vi "M01 Wind Turbine - Dahai.vi"(11 "NXT/EV3":T1) -> (3 "EV3 out":T1)   [LabVIEW 2016]
uses:
  <vilib>/NXT/Subs/LVHSConnector.ctl
  <vilib>/NXT/LegoClasses/BrickReference/BrickReference.lvclass
  <vilib>/NXT/Block Support/NXT_InputPort.ctl
  <vilib>/NXT/Block Support/NXT_OutputPort.ctl
  <vilib>/NXT/Dual Mode Library/Waits/Wait_Num(msec).vi
  <vilib>/NXT/NXTIO Xnodes/NXTIONodeSubVIs/NXTMotorRunDistance.vi
  <vilib>/NXT/NXTIO Xnodes/AddressXNode/NXTIOAddress.xnode
  <vilib>/NXT/NXTIO Xnodes/NXTIOXNode/NXTIO.xnode
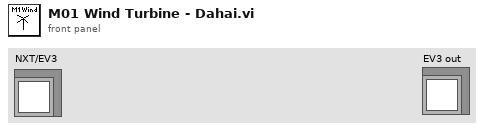
[diagram p1: front panel]
types:
  T1 = typedef "LVHSConnector.ctl" = refnum<class "BrickReference.lvclass">
  T2 = typedef "NXT_OutputPort.ctl" = u8
  T3 = typedef "NXT_InputPort.ctl" = u32
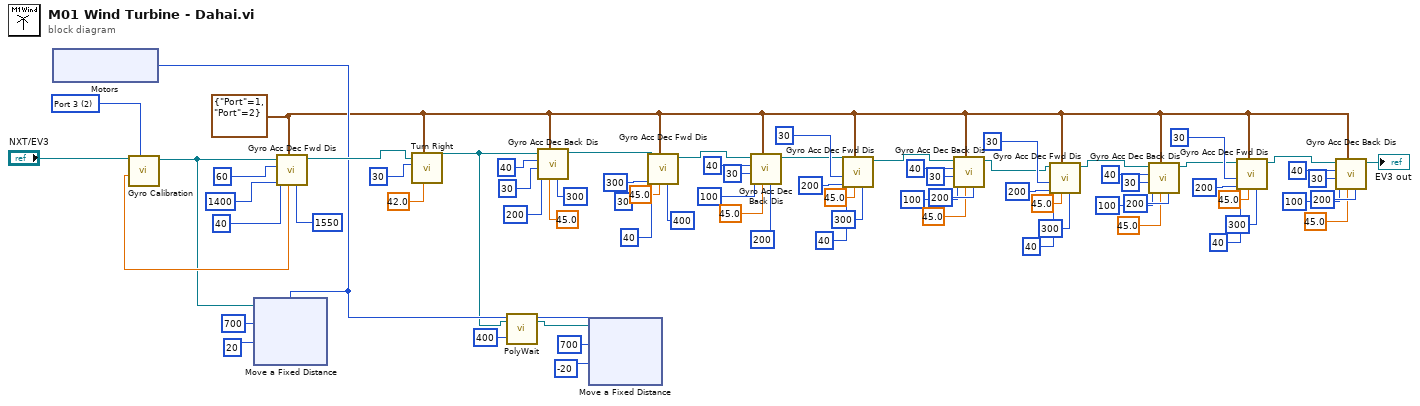
[diagram p0: block diagram]
diagram:
  w2 = cluster{"Port":T2, "Port":T2} {"Port"=1, "Port"=2} ("Motor")
  w74 = T3 2 items=["Port 1", "Port 2", "Port 3", "Port 4"] ("Port (Port 1)")
  n1 = xnode "Motors"() -> ("Motor"=w19:T2)
  n2 = call "Gyro Calibration.vi"("Port (Port 1)"=w74, "NXT/EV3"="NXT/EV3") -> ("Degrees"=w73:sgl, "NXT/EV3"=w23:T1)  [unwired: 5 in, 1 out]
  n3 = xnode "Move a Fixed Distance"("Speed 1"=i8 20, "Distance 1"=700, "Motors"=w19, "NXT/EV3"=w23) -> ()  [unwired: 1 out]
  n4 = call "Gyro Acc Dec Fwd Dis.vi"("Stop rotation"=1550, "Ini. Degrees"=w73, "Motor"=w2, "Threshold to De-acc"=1400, "De-acc"=40, "Acc"=60, "EV3 in"=w23) -> ("EV3 out"=w27:T1)  [unwired: 4 in]
  n5 = call "Turn Right.vi"("Turning angle"=sgl 42.0, "Motor"=w2, "Motor B (right)"=i8 30, "EV3 in"=w27) -> ("EV3 out"=w18:T1)  [unwired: 7 in]
  n6 = call-poly <vilib>:"PolyWait.vi"("Time (100 msec)"=u32 400, "NXT/EV3"=w18) -> ("NXT/EV3"=w17:T1)  [unwired: 2 in]
  n7 = call "Gyro Acc Dec Back Dis.vi"("Stop rotation"=300, "Ini. Degrees"=sgl 45.0, "Motor"=w2, "Threshold to De-acc"=200, "De-acc"=30, "Acc"=40, "EV3 in"=w18) -> ("EV3 out"=w20:T1)  [unwired: 4 in]
  n8 = xnode "Move a Fixed Distance"("Speed 1"=i8 -20, "Distance 1"=700, "Motors"=w19, "NXT/EV3"=w17) -> ()  [unwired: 1 out]
  n9 = call "Gyro Acc Dec Fwd Dis.vi"("Stop rotation"=400, "Ini. Degrees"=sgl 45.0, "Motor"=w2, "Threshold to De-acc"=300, "De-acc"=30, "Acc"=40, "EV3 in"=w20) -> ("EV3 out"=w52:T1)  [unwired: 4 in]
  n10 = call "Gyro Acc Dec Back Dis.vi"("Stop rotation"=200, "Ini. Degrees"=sgl 45.0, "Motor"=w2, "Threshold to De-acc"=100, "De-acc"=30, "Acc"=40, "EV3 in"=w52) -> ("EV3 out"=w40:T1)  [unwired: 4 in]
  n11 = call "Gyro Acc Dec Fwd Dis.vi"("Stop rotation"=300, "Ini. Degrees"=sgl 45.0, "Motor"=w2, "Threshold to De-acc"=200, "De-acc"=30, "Acc"=40, "EV3 in"=w40) -> ("EV3 out"=w51:T1)  [unwired: 4 in]
  n12 = call "Gyro Acc Dec Back Dis.vi"("Stop rotation"=200, "Ini. Degrees"=sgl 45.0, "Motor"=w2, "Threshold to De-acc"=100, "De-acc"=30, "Acc"=40, "EV3 in"=w51) -> ("EV3 out"=w28:T1)  [unwired: 4 in]
  n13 = call "Gyro Acc Dec Fwd Dis.vi"("Stop rotation"=300, "Ini. Degrees"=sgl 45.0, "Motor"=w2, "Threshold to De-acc"=200, "De-acc"=30, "Acc"=40, "EV3 in"=w28) -> ("EV3 out"=w39:T1)  [unwired: 4 in]
  n14 = call "Gyro Acc Dec Back Dis.vi"("Stop rotation"=200, "Ini. Degrees"=sgl 45.0, "Motor"=w2, "Threshold to De-acc"=100, "De-acc"=30, "Acc"=40, "EV3 in"=w39) -> ("EV3 out"=w3:T1)  [unwired: 4 in]
  n15 = call "Gyro Acc Dec Fwd Dis.vi"("Stop rotation"=300, "Ini. Degrees"=sgl 45.0, "Motor"=w2, "Threshold to De-acc"=200, "De-acc"=30, "Acc"=40, "EV3 in"=w3) -> ("EV3 out"=w14:T1)  [unwired: 4 in]
  n16 = call "Gyro Acc Dec Back Dis.vi"("Stop rotation"=200, "Ini. Degrees"=sgl 45.0, "Motor"=w2, "Threshold to De-acc"=100, "De-acc"=30, "Acc"=40, "EV3 in"=w14) -> ("EV3 out"=→"EV3 out":T1)  [unwired: 4 in]
